vi "GetNextTestCase.vi"(0 "TestSeqClass in":refnum<class "TestSeqClass.lvclass">, 11 "error in (no error)":errorcluster) -> (4 "TestSeqClass out":refnum<class "TestSeqClass.lvclass">, 6 "TestMeasureStep.lvclass":refnum<class "TestMeasureStep.lvclass">, 8 "Valid":bool, 10 "Pointer at end":bool, 15 "error out":errorcluster)   [LabVIEW 2017, in "TestSeqClass.lvclass"]
uses:
  TestSeqClass.lvclass
  TestMeasureStep/TestMeasureStep.lvclass
  TestSeqClass.lvclass/TestSeqClass.ctl
  Read CurrentTestPointer.vi
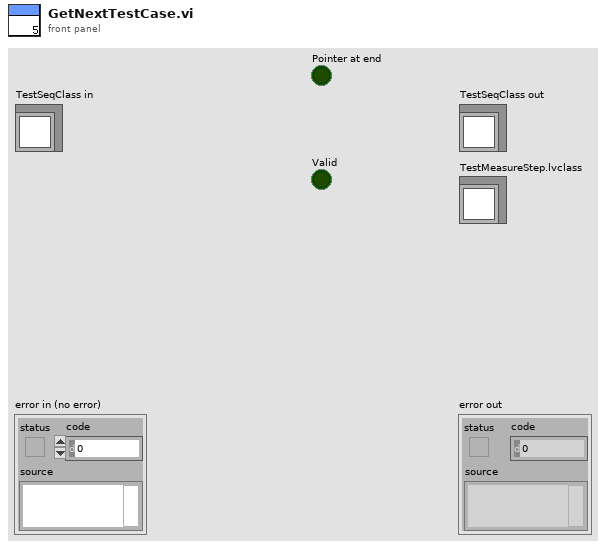
[diagram p1: front panel]
types:
  T1 = typedef "TestSeqType.ctl" = refnum<class "TestMeasureStep.lvclass">[]
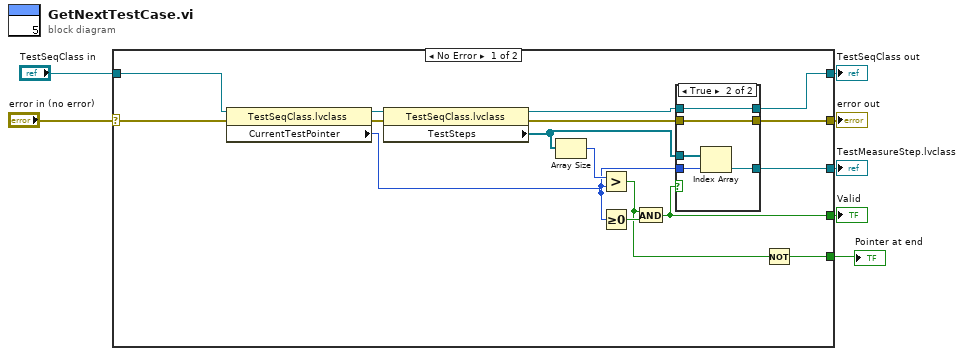
[diagram p0: block diagram]
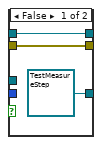
[diagram p2: hidden frame]
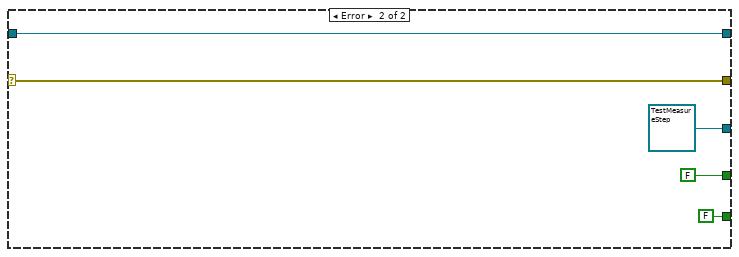
[diagram p3: hidden frame]
diagram:
  n1 = case shown="No Error" "error in (no error)" {
    selector: "error in (no error)" -> [w18 w36]
    tunnel: [w21 w36] -> w6
    tunnel: [w22 w35] -> w4
    tunnel: "TestSeqClass in" -> [w19 w35]
    tunnel: [w20 refnum<class "TestMeasureStep.lvclass"> refnum ("TestMeasureStep.lvclass")] -> w2
    tunnel: [w23 FALSE] -> w3
    tunnel: [w9 FALSE] -> w1
    frame No Error {
      n2 = property class="TestSeqClass.lvclass"(reference=w19, error in=w18) -> (reference out=w17:refnum<class "TestSeqClass.lvclass">, error out=w16:errorcluster, "CurrentTestPointer"=w8:u32)
      n3 = property class="TestSeqClass.lvclass"(reference=w17, error in=w16) -> (reference out=w12:refnum<class "TestSeqClass.lvclass">, error out=w11:errorcluster, "TestSteps"=w13:T1)
      n4 = Array Size(array=w13) -> (size(s)=w15:i32)
      n5 = Greater?(x=w15, y=w8) -> (0:w10:bool)
      n6 = Greater Or Equal To 0?(x=w8) -> (x >= 0?=w14:bool)
      n7 = And(x=w10, y=w14) -> (x .and. y?=w23:bool)
      n8 = case shown="True" w23 {
        tunnel: w13 -> [_ w31]
        tunnel: [refnum<class "TestMeasureStep.lvclass"> refnum ("TestMeasureStep.lvclass") w29] -> w20
        tunnel: w12 -> [w26 w28]
        tunnel: w11 -> [w25 w27]
        tunnel: w8 -> [_ w30]
        tunnel: [w26 w28] -> w22
        tunnel: [w25 w27] -> w21
        frame False {
        }
        frame True {
          n9 = Index Array(array=w31, index=w30) -> (element=w29:refnum<class "TestMeasureStep.lvclass">)
        }
      }
      n10 = Not(x=w10) -> (.not. x?=w9:bool)
    }
    frame Error {
    }
  }
  "error out" <- w6
  "TestSeqClass out" <- w4
  "Valid" <- w3
  "TestMeasureStep.lvclass" <- w2
  "Pointer at end" <- w1
